vi "Read Acceleration.vi"(8 "error in (no error)":errorcluster, 11 "Honeywell Compass HMC6343":refnum<class "Honeywell Compass HMC6343.lvclass">) -> (0 "error out":errorcluster, 2 "Acceleration":cluster{"x (g)":dbl, "y (g)":dbl, "z (g)":dbl}, 3 "Honeywell Compass HMC6343 out":refnum<class "Honeywell Compass HMC6343.lvclass">)   [LabVIEW 2019, in "Honeywell Compass HMC6343.lvclass"]
doc: "Reads Acceleration."
uses:
  Honeywell Compass HMC6343.lvclass
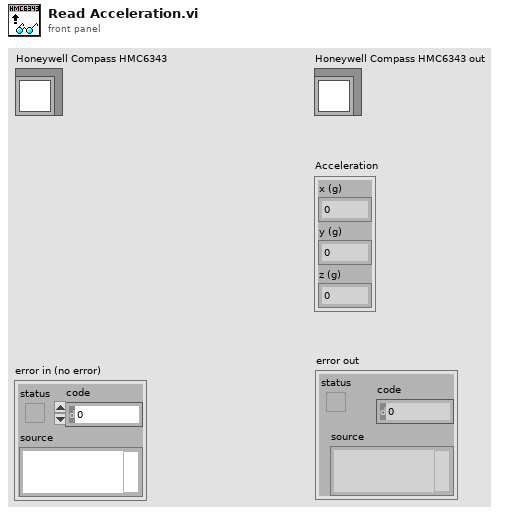
[diagram p1: front panel]
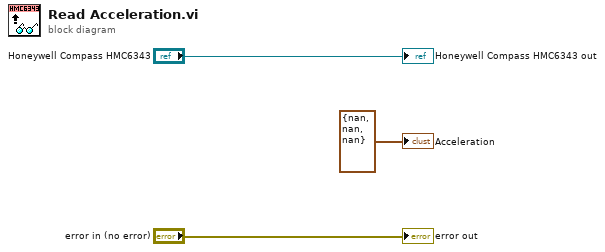
[diagram p0: block diagram]
diagram:
  "error out" <- "error in (no error)"
  "Honeywell Compass HMC6343 out" <- "Honeywell Compass HMC6343"
  "Acceleration" <- cluster{"x (g)":dbl, "y (g)":dbl, "z (g)":dbl} {"x (g)"=nan, "y (g)"=nan, "z (g)"=nan} ("Accel Data")
